vi "Parse Bool Ctl Regs.vi"(8 "APU Registers In":T2, 9 "NTeeths In":T6, 10 "FullyCustomTeeths In":T4, 11 "Boolean":T1[](array[typedef])) -> (0 "APU Registers Out":T2, 1 "NTeeths Out":T6, 2 "FullyCustomTeeths In":T4)   [LabVIEW 2011, in "Engine Sim System Explorer.lvlib"]
uses:
  Engine Sim System Explorer.lvlib
  TypeDefs/NTeethRegs.ctl
  TypeDefs/FullyCustomRegs.ctl
  <userlib>/_FPGA Interface Advanced Tools/FPGA Bitfile Utility/TypeDefs/Scalar Register.ctl
  TypeDefs/APUComp.ctl
  <userlib>/_FPGA Interface Advanced Tools/FPGA Bitfile Utility/FPGA Bitfile Utility.lvlib
panel:
  out "Boolean 2":T1[](array[typedef])
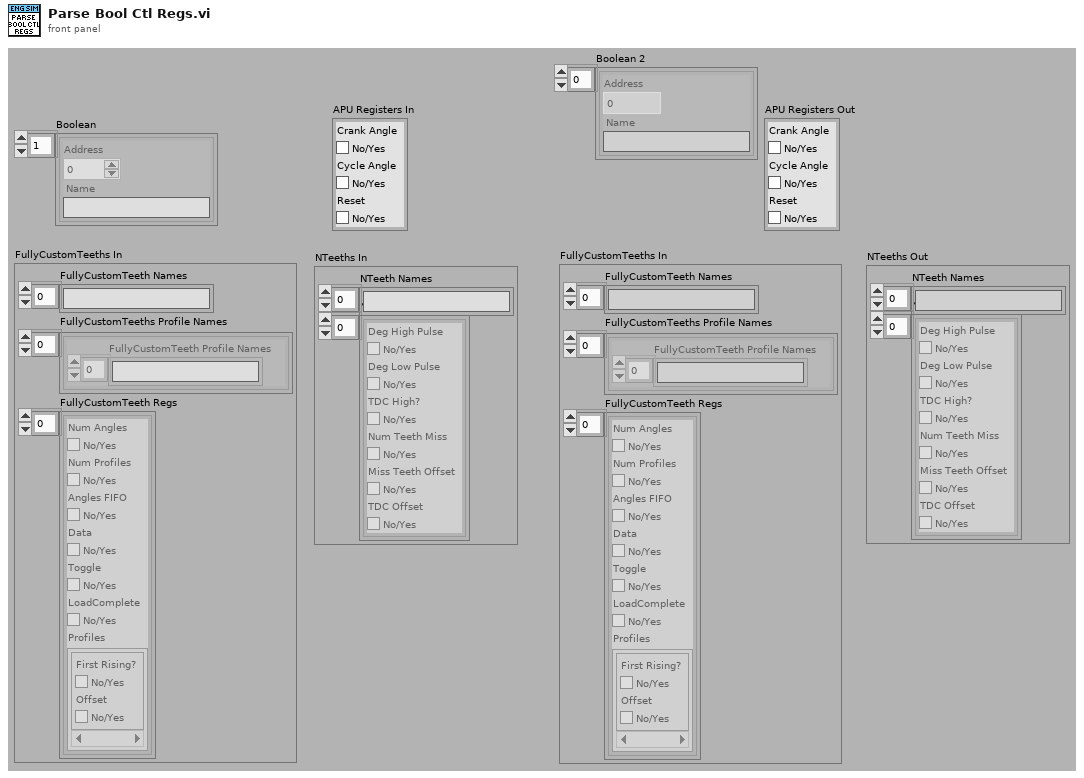
[diagram p1: front panel]
types:
  T1 = typedef "FPGA Bitfile Utility.lvlib/Scalar Register.ctl" = cluster{"Address":u32, "Name":string}
  T2 = typedef "Engine Sim System Explorer.lvlib/APUComp.ctl" = cluster{"Crank Angle":bool, "Cycle Angle":bool, "Reset":bool}
  T3 = typedef "Engine Sim System Explorer.lvlib/FullyCustomRegs.ctl" = cluster{"Num Angles":bool, "Num Profiles":bool, "Angles FIFO":bool, "Data":bool, "Toggle":bool, "LoadComplete":bool, "Profiles":cluster{"First Rising?":bool, "Offset":bool}[]}
  T4 = cluster{"FullyCustomTeeth Names":string[], "FullyCustomTeeths Profile Names":cluster{"FullyCustomTeeth Profile Names":string[]}[], "FullyCustomTeeth Regs":T3[]}
  T5 = typedef "Engine Sim System Explorer.lvlib/NTeethRegs.ctl" = cluster{"Deg High Pulse":bool, "Deg Low Pulse":bool, "TDC High?":bool, "Num Teeth Miss":bool, "Miss Teeth Offset":bool, "TDC Offset":bool}
  T6 = cluster{"NTeeth Names":string[], "NTeeth Regs":T5[]}
  T7 = cluster{"FullyCustomTeeth Profile Names":string[]}
  T8 = cluster{"FullyCustomTeeth Profile Names":string[]}[]
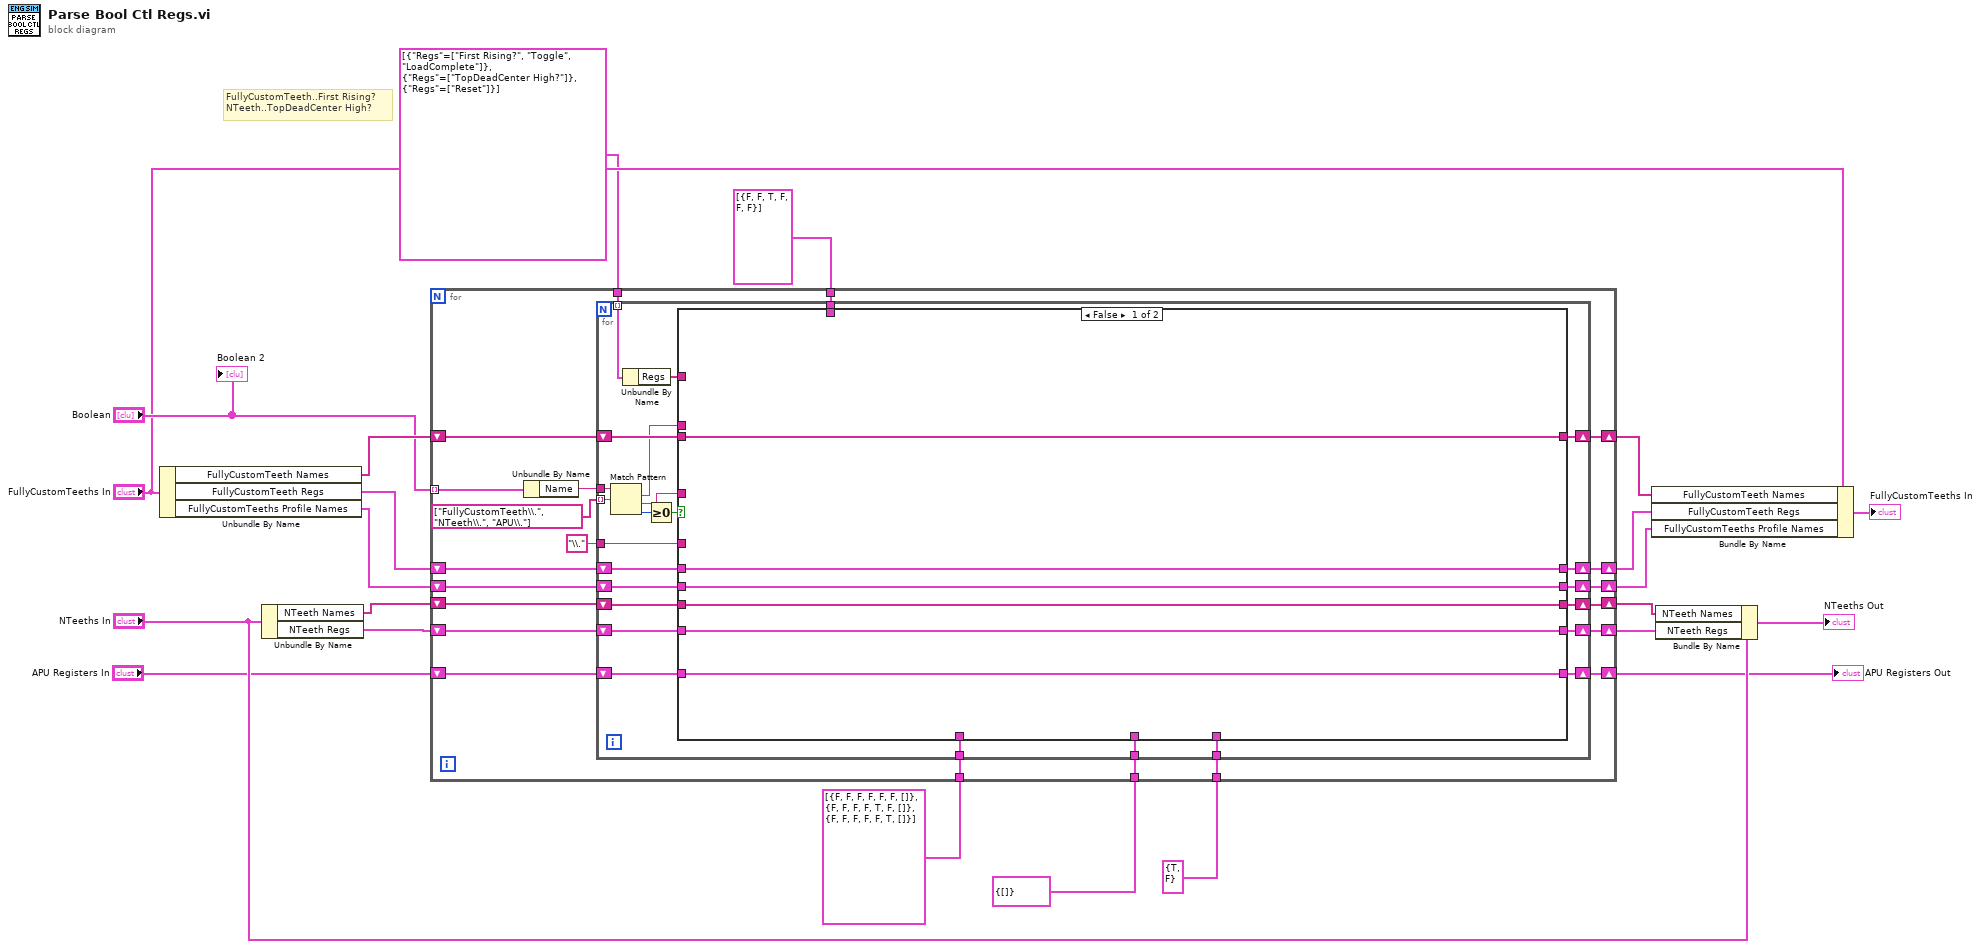
[diagram p0: block diagram]
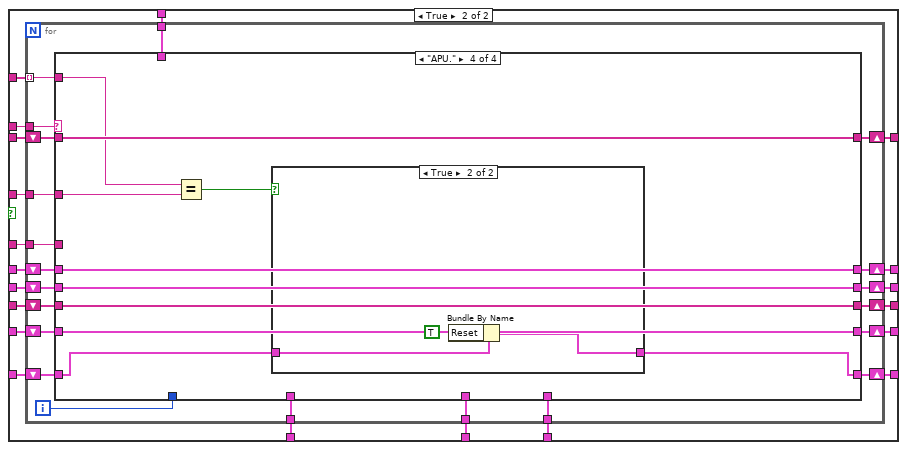
[diagram p2: hidden frame]
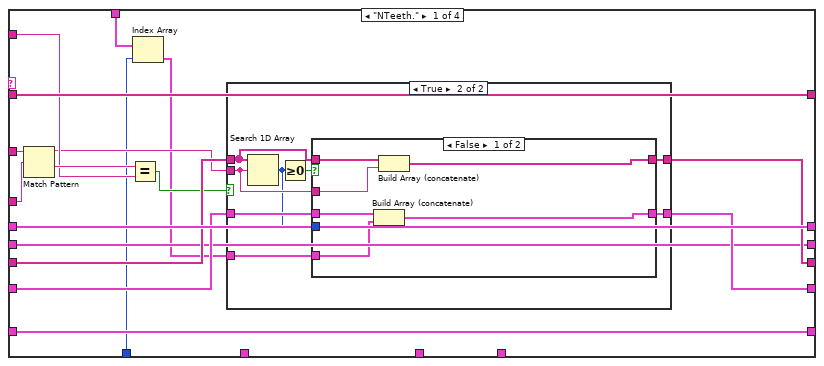
[diagram p3: hidden frame]
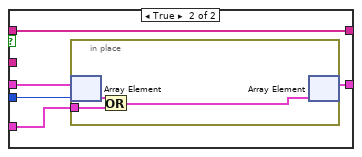
[diagram p5: hidden frame]
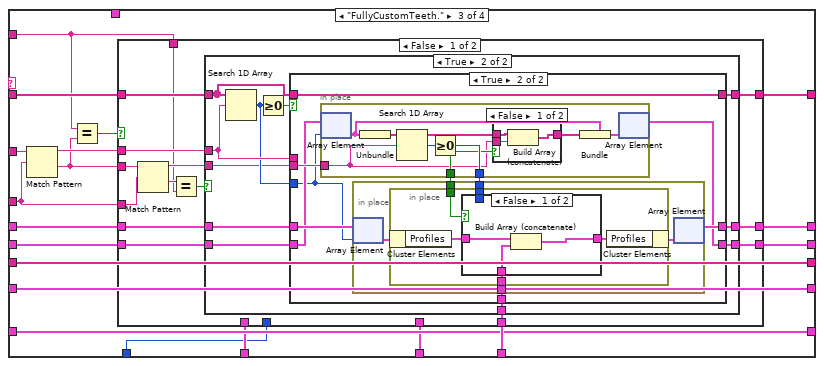
[diagram p7: hidden frame]
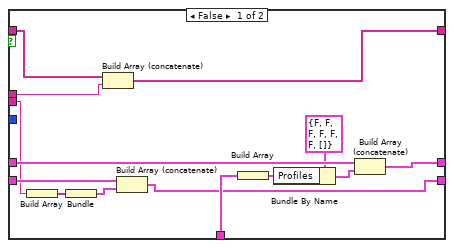
[diagram p9: hidden frame]
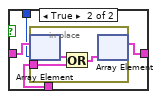
[diagram p11: hidden frame]
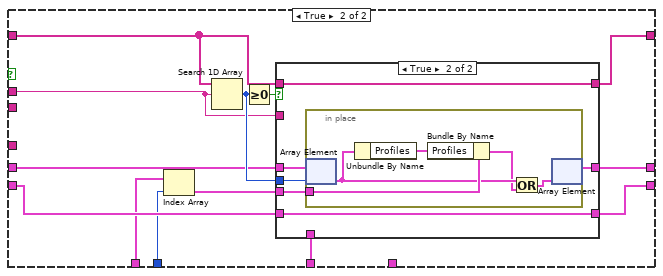
[diagram p12: hidden frame]
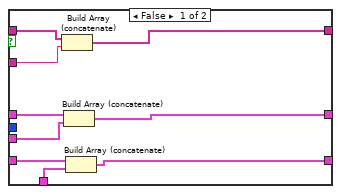
[diagram p13: hidden frame]
diagram:
  # "FullyCustomTeeth..First Rising?\nNTeeth..TopDeadCenter High?"
  n1 = Unbundle By Name("FullyCustomTeeths In") -> ("FullyCustomTeeth Names"=w14:string[], "FullyCustomTeeth Regs"=w15:T3[], "FullyCustomTeeths Profile Names"=w7:T8)
  n2 = Unbundle By Name("NTeeths In") -> ("NTeeth Names"=w16:string[], "NTeeth Regs"=w17:T5[])
  n3 = for {
    tunnel: "Boolean" -> [w43] mode=indexing
    tunnel: cluster{"First Rising?":bool, "Offset":bool} {"First Rising?"=TRUE, "Offset"=FALSE} ("Profile") -> [w41]
    shift-right: [w40] -> w19
    shift-left: w15 -> [w39]
    shift-right: [w38] -> w18
    shift-left: w14 -> [w37]
    tunnel: cluster{"Regs":string[]}[] [{"Regs"=["First Rising?", "Toggle", "LoadComplete"]}, {"Regs"=["TopDeadCenter High?"]}, {"Regs"=["Reset"]}] -> [w35]
    shift-right: [w34] -> w22
    shift-left: w17 -> [w33]
    tunnel: T5[] [{"Deg High Pulse"=FALSE, "Deg Low Pulse"=FALSE, "TDC High?"=TRUE, "Num Teeth Miss"=FALSE, "Miss Teeth Offset"=FALSE, "TDC Offset"=FALSE}] -> [w32]
    shift-right: [w30] -> w21
    shift-left: w16 -> [w29]
    shift-right: [w27] -> w6
    shift-left: w7 -> [w28]
    shift-right: [w25] -> w4
    shift-left: "APU Registers In" -> [w26]
    tunnel: T3[] [{"Num Angles"=FALSE, "Num Profiles"=FALSE, "Angles FIFO"=FALSE, "Data"=FALSE, "Toggle"=FALSE, "LoadComplete"=FALSE, "Profiles"=[]}, {"Num Angles"=FALSE, "Num Profiles"=FALSE, "Angles FIFO"=FALSE, "Data"=FALSE, "Toggle"=TRUE, "LoadComplete"=FALSE, "Profiles"=[]}, {"Num Angles"=FALSE, "Num Profiles"=FALSE, "Angles FIFO"=FALSE, "Data"=FALSE, "Toggle"=FALSE, "LoadComplete"=TRUE, "Profiles"=[]}] -> [w24]
    tunnel: T7 {"FullyCustomTeeth Profile Names"=[]} ("FullyCustomTeeth") -> [w23]
    n4 = Unbundle By Name(w43) -> ("Name"=w42:string)
    n5 = for {
      tunnel: w42 -> [w68]
      tunnel: w41 -> [w64]
      tunnel: string[] ["FullyCustomTeeth\\.", "NTeeth\\.", "APU\\."] -> [w59] mode=indexing
      shift-right: [w61] -> w38
      shift-left: w37 -> [w60]
      shift-right: [w63] -> w40
      shift-left: w39 -> [w62]
      tunnel: w35 -> [w44] mode=indexing
      shift-right: [w56] -> w34
      shift-left: w33 -> [w55]
      tunnel: w32 -> [w54]
      tunnel: "\\." ("regular expression") -> [w53]
      shift-right: [w52] -> w30
      shift-left: w29 -> [w51]
      shift-right: [w49] -> w27
      shift-left: w28 -> [w50]
      shift-right: [w47] -> w25
      shift-left: w26 -> [w48]
      tunnel: w24 -> [w46]
      tunnel: w23 -> [w45]
      n6 = Match Pattern(string=w68, regular expression=w59) -> (match substring=w57:string, after substring=w65:string, offset past match=w67:i32)  [unwired: 1 in, 1 out]
      n7 = Unbundle By Name(w44) -> ("Regs"=w58:string[])
      n8 = Greater Or Equal To 0?(x=w67) -> (x >= 0?=w66:bool)
      n9 = case shown="False" w66 {
        tunnel: w65 -> [_ w94]
        tunnel: w64 -> [_ w93]
        tunnel: [w73 w92] -> w63
        tunnel: w62 -> [w73 w91]
        tunnel: [w74 w90] -> w61
        tunnel: w60 -> [w74 w89]
        tunnel: w58 -> [_ w88]
        tunnel: w57 -> [_ w87]
        tunnel: [w72 w86] -> w56
        tunnel: w55 -> [w72 w85]
        tunnel: w54 -> [_ w84]
        tunnel: w53 -> [_ w83]
        tunnel: [w71 w82] -> w52
        tunnel: w51 -> [w71 w81]
        tunnel: w50 -> [w70 w80]
        tunnel: [w70 w79] -> w49
        tunnel: w48 -> [w69 w78]
        tunnel: [w69 w77] -> w47
        tunnel: w46 -> [_ w76]
        tunnel: w45 -> [_ w75]
        frame False {
        }
        frame True {
          n10 = for {
            tunnel: w94 -> [w104]
            tunnel: w93 -> [w115]
            shift-right: [w112] -> w90
            shift-left: w89 -> [w111]
            shift-right: [w114] -> w92
            shift-left: w91 -> [w113]
            tunnel: w88 -> [w102] mode=indexing
            tunnel: w87 -> [w110]
            shift-right: [w109] -> w86
            shift-left: w85 -> [w107]
            tunnel: w84 -> [w108]
            tunnel: w83 -> [w103]
            shift-right: [w106] -> w82
            shift-left: w81 -> [w105]
            shift-right: [w100] -> w79
            shift-left: w80 -> [w101]
            shift-right: [w98] -> w77
            shift-left: w78 -> [w99]
            tunnel: w76 -> [w97]
            tunnel: w75 -> [w96]
            i -> [w95]
            n11 = case shown="\"APU.\"" w110 {
              tunnel: w104 -> [w125 _ w174 w300]
              tunnel: w115 -> [_ _ w181 _]
              tunnel: [w131 w161 w180 w307] -> w114
              tunnel: w113 -> [w131 w161 w179 w307]
              tunnel: [w132 w162 w178 w303] -> w112
              tunnel: w111 -> [w132 w162 w177 w303]
              tunnel: [w128 w160 w176 w304] -> w109
              tunnel: w108 -> [w117 _ _ _]
              tunnel: w107 -> [w127 w160 w176 w304]
              tunnel: [w129 w159 w175 w305] -> w106
              tunnel: w105 -> [w130 w159 w175 w305]
              tunnel: w103 -> [w124 _ w173 _]
              tunnel: w102 -> [w123 _ w167 w301]
              tunnel: w101 -> [w120 w158 w171 w306]
              tunnel: [w120 w158 w170 w306] -> w100
              tunnel: w99 -> [w119 w157 w169 w299]
              tunnel: [w119 w157 w169 w298] -> w98
              tunnel: w97 -> [_ _ w165 _]
              tunnel: w96 -> [_ _ w164 _]
              tunnel: w95 -> [w118 _ w163 _]
              frame "NTeeth." {
                n12 = Match Pattern(string=w125, regular expression=w124) -> (before substring=w121:string, after substring=w126:string)  [unwired: 1 in, 2 out]
                n13 = Equal?(x=w126, y=w123) -> (x = y?=w122:bool)
                n14 = Index Array(array=w117, index=w118) -> (element=w116:T5)
                n15 = case shown="True" w122 {
                  tunnel: w121 -> [_ w138]
                  tunnel: [w133 w140] -> w128
                  tunnel: w127 -> [w133 w141]
                  tunnel: [w134 w137] -> w129
                  tunnel: w130 -> [w134 w139]
                  tunnel: w116 -> [_ w135]
                  frame False {
                  }
                  frame True {
                    n16 = Search 1D Array(1D array=w139, element=w138) -> (index of element=w136:i32)  [unwired: 1 in]
                    n17 = Greater Or Equal To 0?(x=w136) -> (x >= 0?=w142:bool)
                    n18 = case shown="False" w142 {
                      tunnel: w141 -> [w148 w152]
                      tunnel: w135 -> [w147 w150]
                      tunnel: [w146 w149] -> w140
                      tunnel: w139 -> [w145 w153]
                      tunnel: w138 -> [w144 _]
                      tunnel: [w143 w153] -> w137
                      tunnel: w136 -> [_ w151]
                      frame False {
                        n19 = Build Array (concatenate)(w148, w147) -> (w146:T5[])
                        n20 = Build Array (concatenate)(w145, w144) -> (w143:string[])
                      }
                      frame True {
                        n21 = in-place {
                          in-place-border: w150 -> [w155]
                          n22 = in-place-array #1(w152, w151) -> (w156:T5)
                          n23 = Or(x=w156, y=w155) -> (x .or. y?=w154:T5)
                          n24 = in-place-array #1(w154) -> (w149:T5[])  [unwired: 1 out]
                        }
                      }
                    }
                  }
                }
              }
              frame Default {
              }
              frame "FullyCustomTeeth." {
                n25 = Match Pattern(string=w174, regular expression=w173) -> (before substring=w172:string, after substring=w168:string)  [unwired: 1 in, 2 out]
                n26 = Equal?(x=w167, y=w168) -> (x = y?=w166:bool)
                n27 = case shown="False" w166 {
                  tunnel: w181 -> [w195 _]
                  tunnel: [w194 w269] -> w180
                  tunnel: w179 -> [w193 w273]
                  tunnel: [w192 w270] -> w178
                  tunnel: w177 -> [w191 w275]
                  tunnel: w173 -> [w190 _]
                  tunnel: w172 -> [w189 w274]
                  tunnel: w171 -> [w185 w272]
                  tunnel: [w184 w268] -> w170
                  tunnel: w168 -> [w183 _]
                  tunnel: w167 -> [w182 _]
                  tunnel: w165 -> [_ w267]
                  tunnel: w164 -> [_ w271]
                  tunnel: w163 -> [_ w265]
                  frame False {
                    n28 = Match Pattern(string=w183, regular expression=w190) -> (before substring=w188:string, after substring=w186:string)  [unwired: 1 in, 2 out]
                    n29 = Equal?(x=w186, y=w182) -> (x = y?=w187:bool)
                    n30 = case shown="True" w187 {
                      tunnel: w189 -> [_ w204]
                      tunnel: w195 -> [_ w207]
                      tunnel: [w197 w206] -> w194
                      tunnel: w193 -> [w197 w208]
                      tunnel: [w198 w203] -> w192
                      tunnel: w191 -> [w198 w205]
                      tunnel: w188 -> [_ w199]
                      tunnel: w185 -> [w196 w200]
                      tunnel: [w196 w201] -> w184
                      frame False {
                      }
                      frame True {
                        n31 = Search 1D Array(1D array=w205, element=w204) -> (index of element=w202:i32)  [unwired: 1 in]
                        n32 = Greater Or Equal To 0?(x=w202) -> (x >= 0?=w209:bool)
                        n33 = case shown="True" w209 {
                          tunnel: w208 -> [w223 w232]
                          tunnel: w207 -> [w216 w231]
                          tunnel: [w222 w230] -> w206
                          tunnel: w205 -> [w221 w233]
                          tunnel: w204 -> [w220 _]
                          tunnel: [w219 w233] -> w203
                          tunnel: w202 -> [_ w225]
                          tunnel: [w210 w224] -> w201
                          tunnel: w200 -> [w214 w226]
                          tunnel: w199 -> [w213 w229]
                          frame False {
                            n34 = Build Array(w213) -> (w212:string[])
                            n35 = Bundle(w212) -> (w211:cluster{string[]})  [unwired: 1 in]
                            n36 = Build Array (concatenate)(w221, w220) -> (w219:string[])
                            n37 = Build Array (concatenate)(w214, w211) -> (w210:T8)
                            n38 = Build Array(w216) -> (w215:cluster{"First Rising?":bool, "Offset":bool}[])
                            n39 = Bundle By Name(cluster=T3 {"Num Angles"=FALSE, "Num Profiles"=FALSE, "Angles FIFO"=FALSE, "Data"=FALSE, "Toggle"=FALSE, "LoadComplete"=FALSE, "Profiles"=[]} ("element"), "Profiles"=w215) -> (w218:T3)
                            n40 = Build Array (concatenate)(w223, w218) -> (w222:T3[])
                          }
                          frame True {
                            n41 = in-place {
                              in-place-border: w229 -> [w234]
                              in-place-border: [w237] -> w228
                              in-place-border: [w240] -> w227
                              n42 = in-place-array #2(w226, w225) -> (w239:T7)
                              n43 = Unbundle(w239) -> ("FullyCustomTeeth Profile Names"=w236:string[])
                              n44 = Search 1D Array(1D array=w236, element=w234) -> (index of element=w240:i32)  [unwired: 1 in]
                              n45 = Greater Or Equal To 0?(x=w240) -> (x >= 0?=w237:bool)
                              n46 = case shown="False" w237 {
                                tunnel: w236 -> [w243 w244]
                                tunnel: [w242 w244] -> w235
                                tunnel: w234 -> [w241 _]
                                frame False {
                                n47 = Build Array (concatenate)(w243, w241) -> (w242:string[])
                                }
                                frame True {
                                }
                              }
                              n48 = Bundle(cluster=w239, "FullyCustomTeeth Profile Names"=w235) -> (w238:T7)
                              n49 = in-place-array #2(w238) -> (w224:T8)  [unwired: 1 out]
                            }
                            n50 = in-place {
                              in-place-border: w231 -> [w249]
                              in-place-border: w228 -> [w246]
                              in-place-border: w227 -> [w245]
                              n51 = in-place-array #3(w232, w225) -> (w248:T3)
                              n52 = in-place {
                                in-place-border: w249 -> [w254]
                                in-place-border: w246 -> [w251]
                                in-place-border: w245 -> [w250]
                                n53 = in-place-cluster #4(w248) -> ("Profiles"=w253:cluster{"First Rising?":bool, "Offset":bool}[])
                                n54 = case shown="False" w251 {
                                tunnel: w254 -> [w256 w261]
                                tunnel: w253 -> [w257 w260]
                                tunnel: [w255 w259] -> w252
                                tunnel: w250 -> [_ w258]
                                frame False {
                                n55 = Build Array (concatenate)(w257, w256) -> (w255:cluster{"First Rising?":bool, "Offset":bool}[])
                                }
                                frame True {
                                n56 = in-place {
                                in-place-border: w261 -> [w264]
                                n57 = in-place-array #5(w260, w258) -> (w262:cluster{"First Rising?":bool, "Offset":bool})
                                n58 = Or(x=w262, y=w264) -> (x .or. y?=w263:cluster{"First Rising?":bool, "Offset":bool})
                                n59 = in-place-array #5(w263) -> (w259:cluster{"First Rising?":bool, "Offset":bool}[])  [unwired: 1 out]
                                }
                                }
                                }
                                n60 = in-place-cluster #4("Profiles"=w252) -> (w247:T3)
                              }
                              n61 = in-place-array #3(w247) -> (w230:T3[])  [unwired: 1 out]
                            }
                          }
                        }
                      }
                    }
                  }
                  frame True {
                    n62 = Index Array(array=w267, index=w265) -> (element=w266:T3)
                    n63 = Search 1D Array(1D array=w275, element=w274) -> (index of element=w277:i32)  [unwired: 1 in]
                    n64 = Greater Or Equal To 0?(x=w277) -> (x >= 0?=w276:bool)
                    n65 = case shown="True" w276 {
                      tunnel: w273 -> [w286 w289]
                      tunnel: w266 -> [w285 w287]
                      tunnel: [w284 w290] -> w269
                      tunnel: w275 -> [w283 w292]
                      tunnel: w274 -> [w282 _]
                      tunnel: [w281 w292] -> w270
                      tunnel: w277 -> [_ w288]
                      tunnel: w272 -> [w280 w291]
                      tunnel: [w279 w291] -> w268
                      tunnel: w271 -> [w278 _]
                      frame False {
                        n66 = Build Array (concatenate)(w283, w282) -> (w281:string[])
                        n67 = Build Array (concatenate)(w286, w285) -> (w284:T3[])
                        n68 = Build Array (concatenate)(w280, w278) -> (w279:T8)
                      }
                      frame True {
                        n69 = in-place {
                          in-place-border: w287 -> [w296]
                          n70 = in-place-array #6(w289, w288) -> (w295:T3)
                          n71 = Unbundle By Name(w295) -> ("Profiles"=w294:cluster{"First Rising?":bool, "Offset":bool}[])
                          n72 = Bundle By Name(cluster=w296, "Profiles"=w294) -> (w293:T3)
                          n73 = Or(x=w295, y=w293) -> (x .or. y?=w297:T3)
                          n74 = in-place-array #6(w297) -> (w290:T3[])  [unwired: 1 out]
                        }
                      }
                    }
                  }
                }
              }
              frame "APU." {
                n75 = Equal?(x=w301, y=w300) -> (x = y?=w302:bool)
                n76 = case shown="True" w302 {
                  tunnel: w299 -> [w308 w311]
                  tunnel: [w308 w310] -> w298
                  frame False {
                  }
                  frame True {
                    n77 = Bundle By Name(cluster=w311, "Reset"=TRUE) -> (w310:T2)
                  }
                }
              }
            }
          }
        }
      }
    }
  }
  "APU Registers Out" <- w4
  n78 = Bundle By Name(cluster="FullyCustomTeeths In", "FullyCustomTeeth Names"=w18, "FullyCustomTeeth Regs"=w19, "FullyCustomTeeths Profile Names"=w6) -> (→"FullyCustomTeeths In":T4)
  n79 = Bundle By Name(cluster="NTeeths In", "NTeeth Names"=w21, "NTeeth Regs"=w22) -> (→"NTeeths Out":T6)
  "Boolean 2" <- "Boolean"
